vi "Handle Messages.vi"(8 "error in (no error)":errorcluster, 9 "Message Data":variant, 10 "Message":string, 11 "Work Dispatcher In":refnum<class "Work Dispatcher.lvclass">) -> (0 "error out":errorcluster, 3 "Work Dispatcher Out":refnum<class "Work Dispatcher.lvclass">)   [LabVIEW 2020, in "Work Dispatcher.lvclass"]
uses:
  Work Dispatcher.lvclass
  C:/Program Files (x86)/National Instruments/LabVIEW 2020/vi.lib/Asteme/Triarc Framework/Helper Loop/Helper Loop.lvclass
  Process Job/Job Handler.lvclass
  Work Dispatcher.lvclass/Work Dispatcher.ctl
  <vilib>/Asteme/Triarc Framework/Process/Process.lvclass
  <vilib>/Asteme/Triarc Framework/Helper Loop/Helper Loop.lvclass
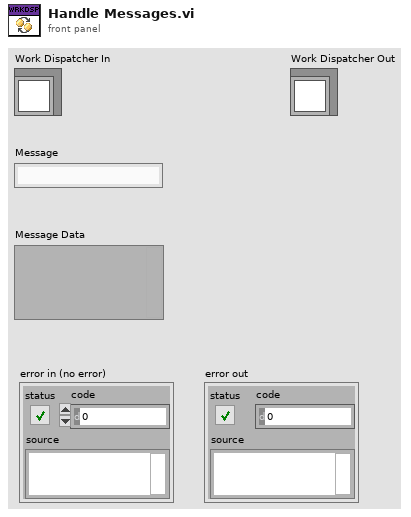
[diagram p1: front panel]
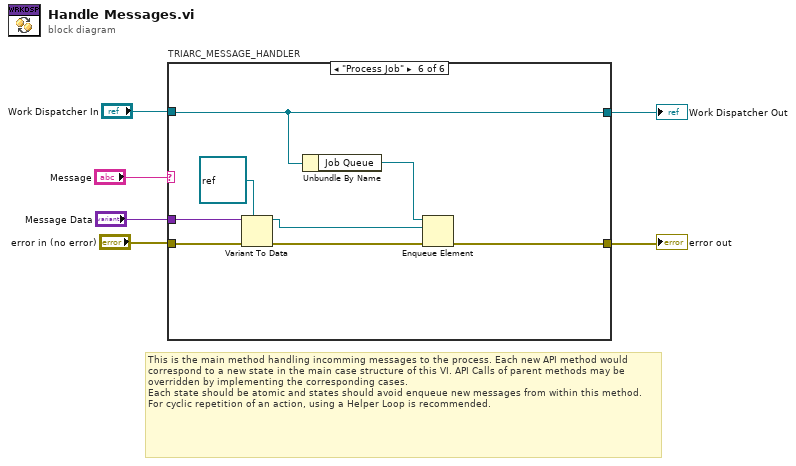
[diagram p0: block diagram]
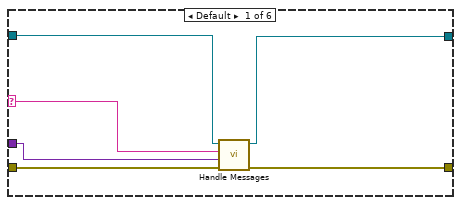
[diagram p2: hidden frame]
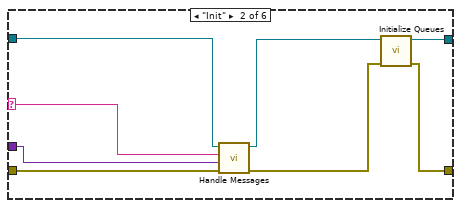
[diagram p3: hidden frame]
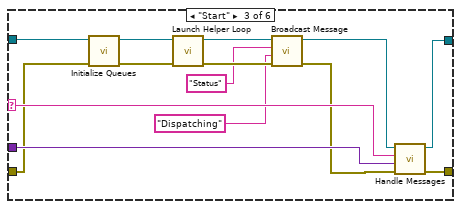
[diagram p4: hidden frame]
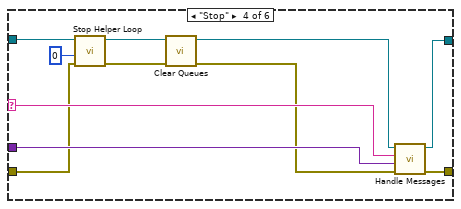
[diagram p5: hidden frame]
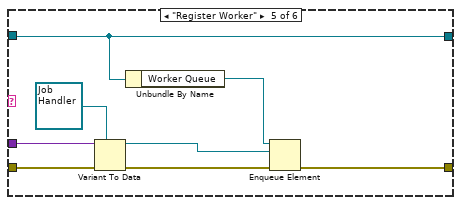
[diagram p6: hidden frame]
diagram:
  # "This is the main method handling incomming messages to the process. Each new API method would correspond to a new state in the main case structure of this VI. API Calls of parent methods may be overridden by implementing the corresponding cases.\nEach state should be atomic and states should avoid enqueue new messages from within this method. For cyclic repetition of an action, using a Helper Loop is recommended."
  n1 = case "TRIARC_MESSAGE_HANDLER" shown="\"Process Job\"" "Message" {
    selector: "Message" -> [w10 w18 w32 w44 _ _]
    tunnel: "error in (no error)" -> [w9 w17 w31 w36 w53 w61]
    tunnel: "Work Dispatcher In" -> [w12 w20 w34 w40 w49 w56]
    tunnel: "Message Data" -> [w11 w19 w33 w45 w51 w58]
    tunnel: [w8 w13 w30 w43 w48 w57] -> w2
    tunnel: [w7 w15 w29 w42 w49 w56] -> w1
    frame Default {
      n2 = call-parent "Handle Messages.vi"("error in (no error)"=w9, "Message Data"=w11, "Message"=w10, "Process In"=w12) -> ("error out"=w8:errorcluster, "Process Out"=w7:refnum<class "Work Dispatcher.lvclass">)  [unwired: 6 in]
    }
    frame "Init" {
      n3 = call-parent "Handle Messages.vi"("error in (no error)"=w17, "Message Data"=w19, "Message"=w18, "Process In"=w20) -> ("error out"=w14:errorcluster, "Process Out"=w16:refnum<class "Work Dispatcher.lvclass">)  [unwired: 6 in]
      n4 = call "Initialize Queues.vi"("error in (no error)"=w14, "Work Dispatcher in"=w16) -> ("error out"=w13:errorcluster, "Work Dispatcher out"=w15:refnum<class "Work Dispatcher.lvclass">)  [unwired: 8 in]
    }
    frame "Start" {
      n5 = call "Initialize Queues.vi"("error in (no error)"=w31, "Work Dispatcher in"=w34) -> ("error out"=w28:errorcluster, "Work Dispatcher out"=w26:refnum<class "Work Dispatcher.lvclass">)  [unwired: 8 in]
      n6 = call <vilib>:"Launch Helper Loop.vi"("error in (no error)"=w28, "Helper Loop In"=w26) -> ("error out"=w27:errorcluster, "Helper Loop Out"=w24:refnum<class "Work Dispatcher.lvclass">)  [unwired: 8 in]
      n7 = call-dynamic "Broadcast Message.vi"("error in (no error)"=w27, "Message Data"="Dispatching" ("Message"), "Message"="Status", "Rig Process In"=w24) -> ("error out"=w25:errorcluster, "Rig Process Out"=w23:refnum<class "Work Dispatcher.lvclass">)  [unwired: 6 in]
      n8 = call-parent "Handle Messages.vi"("error in (no error)"=w25, "Message Data"=w33, "Message"=w32, "Process In"=w23) -> ("error out"=w30:errorcluster, "Process Out"=w29:refnum<class "Work Dispatcher.lvclass">)  [unwired: 6 in]
    }
    frame "Stop" {
      n9 = call <vilib>:"Stop Helper Loop.vi"("error in (no error)"=w36, "timeout in ms (-1)"=0, "Helper Loop In"=w40) -> ("error out"=w37:errorcluster, "Helper Loop Out"=w38:refnum<class "Work Dispatcher.lvclass">)  [unwired: 6 in, 1 out]
      n10 = call "Clear Queues.vi"("error in (no error)"=w37, "Work Dispatcher in"=w38) -> ("error out"=w41:errorcluster, "Work Dispatcher out"=w39:refnum<class "Work Dispatcher.lvclass">)  [unwired: 8 in]
      n11 = call-parent "Handle Messages.vi"("error in (no error)"=w41, "Message Data"=w45, "Message"=w44, "Process In"=w39) -> ("error out"=w43:errorcluster, "Process Out"=w42:refnum<class "Work Dispatcher.lvclass">)  [unwired: 6 in]
    }
    frame "Register Worker" {
      n12 = Variant To Data(error in=w53, type=refnum<class "Job Handler.lvclass"> refnum ("Process Job.lvclass"), Variant=w51) -> (data=w46:refnum<class "Job Handler.lvclass">, error out=w52:errorcluster)
      n13 = Unbundle By Name(w49) -> ("Worker Queue"=w47:refnum<queue>)
      n14 = Enqueue Element(queue=w47, element=w46, error in (no error)=w52) -> (error out=w48:errorcluster)  [unwired: 1 in, 2 out]
    }
    frame "Process Job" {
      n15 = Variant To Data(error in=w61, type=refnum<class> refnum ("LabVIEW Object"), Variant=w58) -> (data=w54:refnum<class>, error out=w60:errorcluster)
      n16 = Unbundle By Name(w56) -> ("Job Queue"=w55:refnum<queue>)
      n17 = Enqueue Element(queue=w55, element=w54, error in (no error)=w60) -> (error out=w57:errorcluster)  [unwired: 1 in, 2 out]
    }
  }
  "error out" <- w2
  "Work Dispatcher Out" <- w1
